vi "GetErrorType.vi"(10 "error in (no error)":errorcluster) -> (2 "ErrorType":T1)   [LabVIEW 2017, in "Transparent Assertions.lvlib" / "Constraints.lvlib" / "Error.lvclass"]
uses:
  Error.lvclass
  ErrorType.ctl
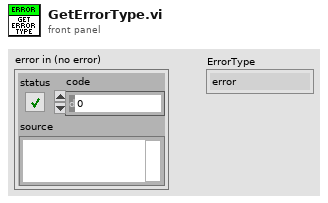
[diagram p1: front panel]
types:
  T1 = typedef "Transparent Assertions.lvlib/Constraints.lvlib/Error.lvclass/ErrorType.ctl" = enum16{"error", "warning", "no error"}
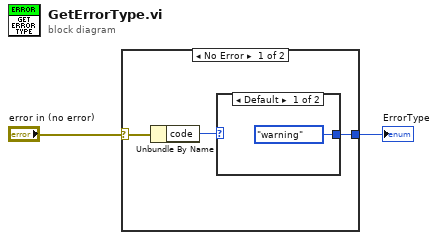
[diagram p0: block diagram]
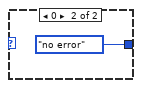
[diagram p2: hidden frame]
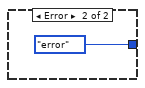
[diagram p3: hidden frame]
diagram:
  n1 = case shown="No Error" "error in (no error)" {
    selector: "error in (no error)" -> [w4 _]
    tunnel: [w5 ErrorType."error" ("ErrorType")] -> w1
    frame No Error {
      n2 = Unbundle By Name(w4) -> ("code"=w3:i32)
      n3 = case shown="Default" w3 {
        tunnel: [ErrorType."warning" ("ErrorType") ErrorType."no error" ("ErrorType")] -> w5
        frame Default {
        }
        frame 0 {
        }
      }
    }
    frame Error {
    }
  }
  "ErrorType" <- w1
